vi "Get Variable Name List.vi"(7 "Target (Process)":T1 items=["Process", "User", "Machine"], 8 "Error In":errorcluster) -> (0 "Error Out":errorcluster, 3 "Names[]":string[](array[string]))   [LabVIEW 2023, in "SLL Environment Variable.lvlib"]
doc: "Get the list of environment variables in the target environment."
uses:
  SLL Environment Variable.lvlib
  _Typedef/Target Environment Enum.ctl
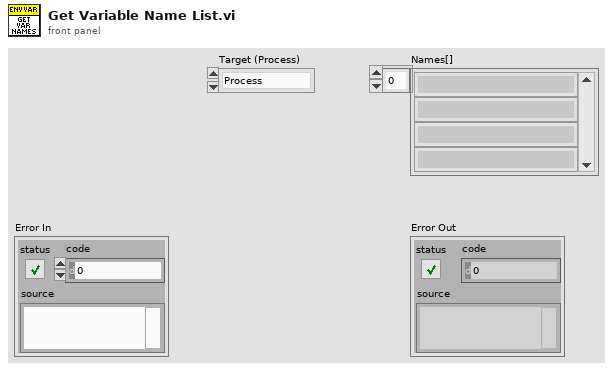
[diagram p1: front panel]
types:
  T1 = typedef "SLL Environment Variable.lvlib/Target Environment Enum.ctl" = i32
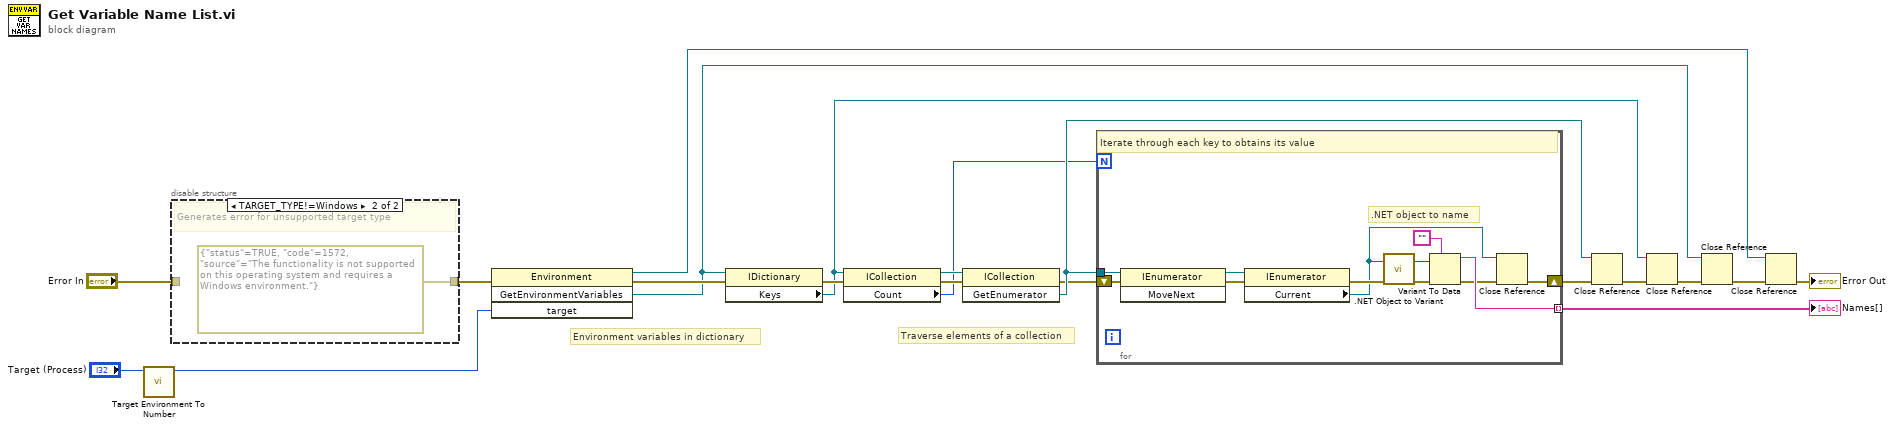
[diagram p0: block diagram]
diagram:
  # "Traverse elements of a collection"
  # "Environment variables in dictionary"
  n1 = call "Target Environment To Number.vi"("Target (Process)"="Target (Process)") -> ("Number"=w3:i32)  [unwired: 10 in]
  n2 = disable-structure shown="TARGET_TYPE!=Windows" {
    disable-tunnel: "Error In" -> [w21 _]
    disable-tunnel: [w21 errorcluster {"status"=TRUE, "code"=1572, "source"="The functionality is not supported on this operating system and requires a Windows environment."} ("Error In")] -> w2
    frame condition #0 (active) {
    }
    frame condition #1 {
      # "Generates error for unsupported target type"
    }
  }
  n3 = invoke class="Environment" method="GetEnvironmentVariables"(error in=w2, "target"=w3) -> (reference out=w8:refnum<k24>, error out=w11:errorcluster, "GetEnvironmentVariables"=w10:refnum<k24>)  [unwired: 2 in, 1 out]
  n4 = property class="IDictionary"(reference=w10, error in=w11) -> (error out=w12:errorcluster, "Keys"=w7:refnum<k24>)  [unwired: 1 out]
  n5 = property class="ICollection"(reference=w7, error in=w12) -> (reference out=w14:refnum<k24>, error out=w13:errorcluster, "Count"=w6:i32)
  n6 = invoke class="ICollection" method="GetEnumerator"(reference=w14, error in=w13) -> (error out=w15:errorcluster, "GetEnumerator"=w16:refnum<k24>)  [unwired: 1 in, 1 out]
  n7 = for {
    N: w6 -> [_]
    tunnel: w16 -> [w30]
    tunnel: [w33] -> w5 mode=indexing
    shift-right: [w32] -> w20
    shift-left: w15 -> [w34]
    # ".NET object to name"
    # "Iterate through each key to obtains its value"
    n8 = invoke class="IEnumerator" method="MoveNext"(reference=w30, error in=w34) -> (reference out=w23:refnum<k24>, error out=w31:errorcluster)  [unwired: 1 in, 1 out]
    n9 = property class="IEnumerator"(reference=w23, error in=w31) -> (error out=w29:errorcluster, "Current"=w24:refnum<k24>)  [unwired: 1 out]
    n10 = call <vilib>:".NET Object to Variant.vi"("error in (no error)"=w29, ".NET object"=w24) -> ("error out"=w28:errorcluster, "variant"=w27:variant)
    n11 = Variant To Data(error in=w28, type="", Variant=w27) -> (data=w33:string, error out=w26:errorcluster)
    n12 = Close Reference(reference=w24, error in (no error)=w26) -> (error out=w32:errorcluster)
  }
  "Names[]" <- w5
  n13 = Close Reference(reference=w16, error in (no error)=w20) -> (error out=w17:errorcluster)
  n14 = Close Reference(reference=w7, error in (no error)=w17) -> (error out=w18:errorcluster)
  n15 = Close Reference(reference=w10, error in (no error)=w18) -> (error out=w19:errorcluster)
  n16 = Close Reference(reference=w8, error in (no error)=w19) -> (error out=→"Error Out":errorcluster)
